vi "Calculator.vi"() -> ()   [LabVIEW 2014]
doc: "This VI is a fully-functional calculator built in LabVIEW. It demonstrates the following concepts taught in the LabVIEW Basics class.\n\n- Dataflow Programming\n- Modular Programming\n- While Loops\n- Shift Registers\n- Case Structures\n- Functional Global Variables\n- Event-Driven Programming\n- VI Documentation\n- Control/Indicator Documentation\n- Custom Controls/Type Definitions\n- LabVIEW Project and Application Builder\n\nAuthor: Erik Johnson, National Instruments"
uses:
  Custom Controls/Operation Buttons.ctl
  Custom Controls/Memory Options.ctl
panel:
  in  "Memory Add":bool
  in  "Memory Store":bool
  in  "Memory Recall":bool
  in  "Memory Clear":bool
  in  "Decimal":bool
  in  "Inverse":bool
  in  "Squared":bool
  in  "Square Root":bool
  in  "Negate":bool
  in  "error in (no error)":errorcluster
  in  "Backspace":bool
  in  "Clear All":bool
  in  "Clear Entry":bool
  in  "Display":ext format="%#_15f"
  in  "Equals":bool
  in  "Divide":bool
  in  "Multiply":bool
  in  "Subtract":bool
  in  "Add":bool
  in  "Zero":bool
  in  "Nine":bool
  in  "Eight":bool
  in  "Seven":bool
  in  "Six":bool
  in  "Five":bool
  in  "Four":bool
  in  "Three":bool
  in  "Two":bool
  in  "One":bool
  # "M"
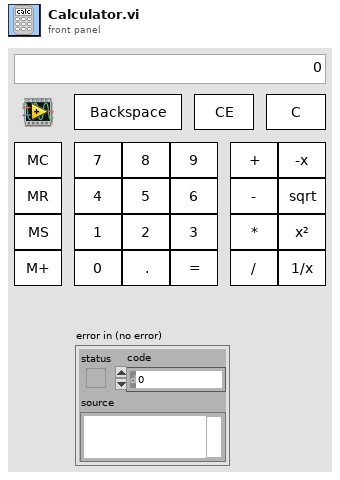
[diagram p1: front panel]
types:
  T1 = typedef "Operation Buttons.ctl" = enum16{"Add", "Subtract", "Multiply", "Divide", "Equals"}
  T2 = typedef "Memory Options.ctl" = enum16{"Memory Clear", "Memory Recall", "Memory Store", "Memory Add"}
  T3 = enum32{"invalid app kind", "Development System", "Run Time System", "Student Edition", "Embedded LabVIEW", "Evaluation", "Custom"}
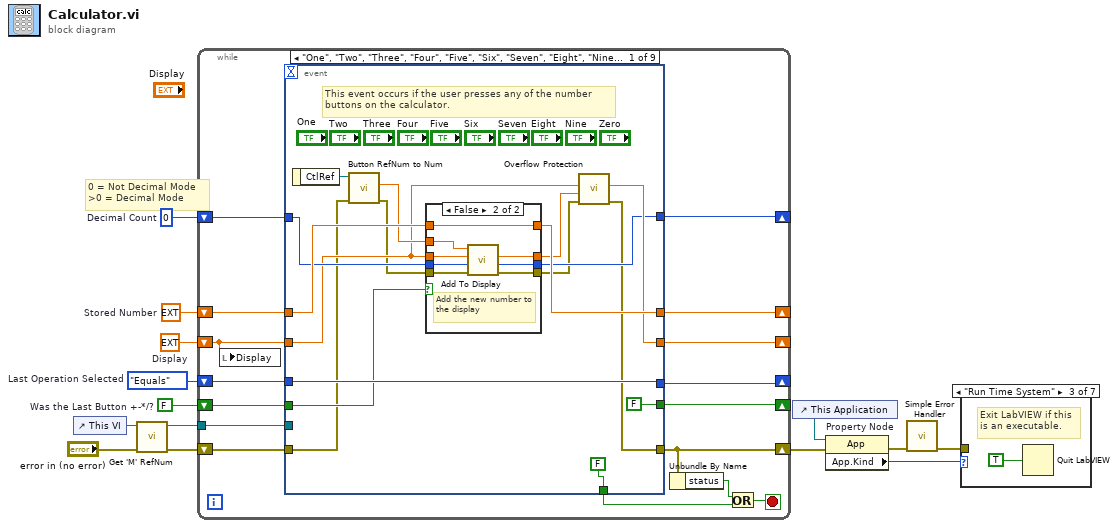
[diagram p0: block diagram]
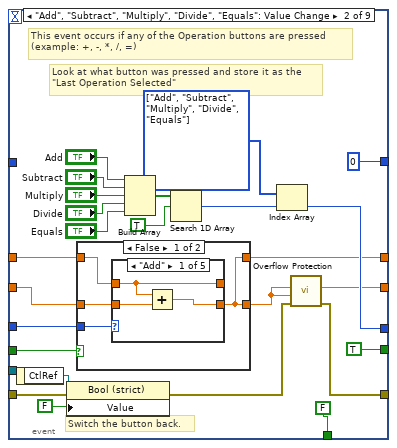
[diagram p9: hidden frame]
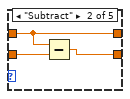
[diagram p10: hidden frame]
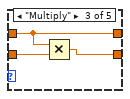
[diagram p11: hidden frame]
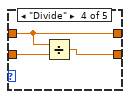
[diagram p12: hidden frame]
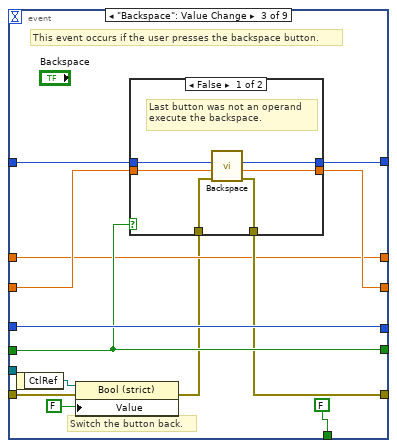
[diagram p15: hidden frame]
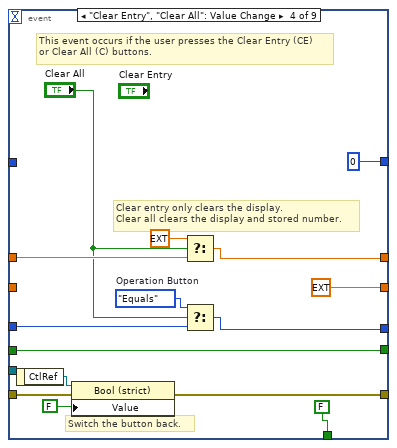
[diagram p17: hidden frame]
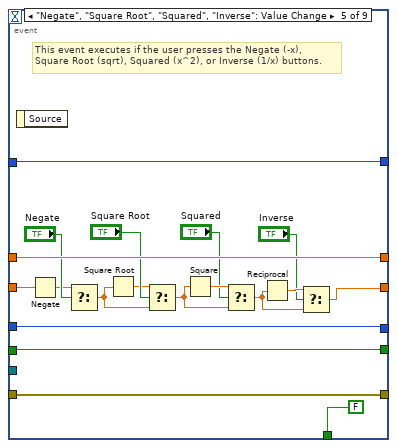
[diagram p18: hidden frame]
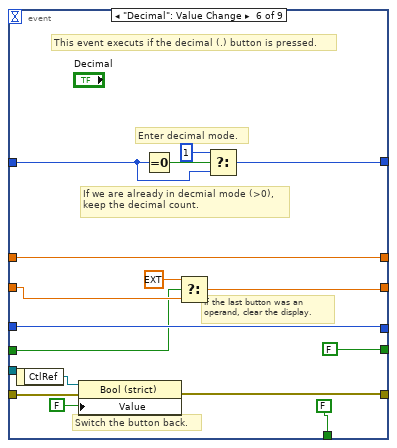
[diagram p19: hidden frame]
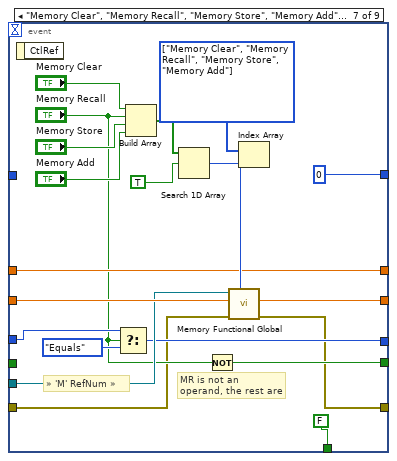
[diagram p20: hidden frame]
diagram:
  w8 = u8 0  # Decimal Count
  w9 = Operation_Buttons."Equals"  # Last Operation Selected
  w12 = FALSE  # Was the Last Button +-*/?
  w13 = ext 0.0  # Stored Number
  w14 = ext 0.0  # Display
  # "0 = Not Decimal Mode\n>0 = Decimal Mode"
  n1 = control-ref of="This VI"() -> (w7:refnum<vi>)
  n2 = call "Get 'M' RefNum.vi"("error in (no error)"="error in (no error)", "This VI"=w7) -> ("error out"=w5:errorcluster, "'M' Refnum"=w6:refnum<vi>)  [unwired: 8 in]
  n3 = while {
    shift-right: [w29] -> _
    shift-left: w14 -> [w30]
    shift-right: [w20] -> _
    shift-left: w13 -> [w28]
    shift-right: [w26] -> _
    shift-left: w9 -> [w27]
    shift-right: [w24] -> _
    shift-left: w12 -> [w25]
    shift-right: [w22] -> _
    shift-left: w8 -> [w23]
    tunnel: w6 -> [w21]
    shift-right: [w17] -> w2
    shift-left: w5 -> [w19]
    stop <- w18 stop-if-true
    n4 = local write "Display"(w30) -> ()
    n5 = event shown="[0] \"One\", \"Two\", \"Three\", \"Four\", \"Five\", \"Six\", \"Seven\", \"Eight\", \"Nine\", \"Zero\": Value Change" {
      selector: _ -> [_ _ _ _ _ _ _ _ _]
      dyn-events: _ -> [_ _ _ _ _ _ _ _ _]
      timeout: _ -> [_ _ _ _ _ _ _ _ _]
      tunnel: [w44 w63 w115 ext 0.0 ("Display") w148 w163 w189 w201 0.0 ("Display")] -> w29
      tunnel: w30 -> [w38 w83 w116 _ w156 w164 w190 w201 _]
      tunnel: [FALSE ("Discard?") FALSE ("Discard?") FALSE ("Discard?") FALSE ("Discard?") FALSE ("Discard?") FALSE ("Discard?") FALSE ("Discard?") FALSE ("Discard?") TRUE ("Discard?")] -> w15
      tunnel: w28 -> [w43 w84 w109 w138 w160 w175 w188 w202 _]
      tunnel: [w45 w62 w109 w137 w160 w175 w188 w202 ext 0.0 ("Stored Number")] -> w20
      tunnel: w27 -> [w37 w74 w117 w132 w159 w176 w185 w205 _]
      tunnel: [w37 w66 w117 w131 w159 w176 w182 w205 w268] -> w26
      tunnel: w25 -> [w36 w72 w114 w141 w144 w161 _ w206 _]
      tunnel: [FALSE ("Discard?") TRUE ("Discard?") w114 w141 w144 FALSE ("Discard?") w180 w206 FALSE ("Discard?")] -> w24
      tunnel: w23 -> [w42 _ w113 _ w143 w173 _ w203 _]
      tunnel: [w41 u8 0 ("Decimal Count") w112 u8 0 ("Decimal Count") w143 w171 u8 0 ("Decimal Count") w203 u8 0 ("Decimal Count")] -> w22
      tunnel: w21 -> [_ _ _ _ _ _ w186 _ _]
      tunnel: w19 -> [w35 w67 w108 w129 w142 w168 w178 w199 w266]
      tunnel: [w32 w60 w110 w128 w142 w167 w177 w198 w266] -> w17
      event "One", "Two", "Three", "Four", "Five", "Six", "Seven", "Eight", "Nine", "Zero": Value Change {
        # "This event occurs if the user presses any of the number\nbuttons on the calculator."
        n6 = event-data() -> ("CtlRef"=w31:refnum<vi>)  [unwired: 1 in]
        n7 = call "Button RefNum to Num.vi"("error in (no error)"=w35, "Button Reference"=w31) -> ("error out"=w34:errorcluster, "Number on Button"=w40:dbl)  [unwired: 8 in]
        n8 = case shown="False" w36 {
          tunnel: w38 -> [w51 w55]
          tunnel: [w49 w54] -> w39
          tunnel: w43 -> [_ w59]
          tunnel: [w51 w59] -> w45
          tunnel: w42 -> [w50 w57]
          tunnel: [w50 w58] -> w41
          tunnel: w40 -> [w49 w56]
          tunnel: w34 -> [w48 w53]
          tunnel: [w48 w52] -> w33
          frame True {
            # "Last button was an operand, refresh the display."
          }
          frame False {
            # "Add the new number to the display"
            n9 = call "Add To Display.vi"("error in (no error)"=w53, "Decimal Count In"=w57, "Display In"=w55, "Number In"=w56) -> ("error out"=w52:errorcluster, "Decimal Count Out"=w58:u8, "Display Out"=w54:ext)  [unwired: 5 in]
          }
        }
        n10 = call "Overflow Protection.vi"("error in (no error)"=w33, "Display After"=w39, "Display Before"=w38) -> ("error out"=w32:errorcluster, "Display Output"=w44:ext)  [unwired: 7 in]
      }
      event "Add", "Subtract", "Multiply", "Divide", "Equals": Value Change {
        w71 = T1[] [enum."Add", enum."Subtract", enum."Multiply", enum."Divide", enum."Equals"] items=["Add", "Subtract", "Multiply", "Divide", "Equals"]
        # "Switch the button back."
        # "Look at what button was pressed and store it as the\n\"Last Operation Selected\""
        # "This event occurs if any of the Operation buttons are pressed\n(example: +, -, *, /, =)"
        n11 = event-data() -> ("CtlRef"=w69:refnum<vi>)  [unwired: 1 in]
        n12 = property class="Bool (strict)"(reference=w69, error in=w67, "Value"=FALSE) -> (error out=w61:errorcluster)  [unwired: 1 out]
        n13 = case shown="False" w72 {
          tunnel: w84 -> [w88 w103]
          tunnel: w83 -> [w87 w104]
          tunnel: w74 -> [w85 _]
          tunnel: [w86 w104] -> w64
          tunnel: [w86 w103] -> w62
          frame False {
            n14 = case shown="\"Add\"" w85 {
              tunnel: w88 -> [w89 w92 w95 w98 w101]
              tunnel: w87 -> [w91 w94 w97 w100 w102]
              tunnel: [w90 w93 w96 w99 w102] -> w86
              tunnel: [w89 w92 w95 w98 w101] -> _
              frame "Add" {
                n15 = Add(x=w89, y=w91) -> (x+y=w90:ext)
              }
              frame "Subtract" {
                n16 = Subtract(x=w92, y=w94) -> (x-y=w93:ext)
              }
              frame "Multiply" {
                n17 = Multiply(x=w95, y=w97) -> (x*y=w96:ext)
              }
              frame "Divide" {
                n18 = Divide(x=w98, y=w100) -> (x/y=w99:ext)
              }
              frame "Equals", Default {
              }
            }
          }
          frame True {
            # "If the last button was an operation, overwrite it and throw out the previous operation."
          }
        }
        n19 = Build Array "Build Array"("Add", "Subtract", "Multiply", "Divide", "Equals") -> (w77:bool[])
        n20 = Search 1D Array(1D array=w77, element=TRUE) -> (index of element=w75:i32)  [unwired: 1 in]
        n21 = Index Array "Index Array"(array=w71, index=w75) -> (element=w66:T1)
        n22 = call "Overflow Protection.vi"("error in (no error)"=w61, "Display After"=w64, "Display Before"=w64) -> ("error out"=w60:errorcluster, "Display Output"=w63:ext)  [unwired: 7 in]
      }
      event "Backspace": Value Change {
        # "Switch the button back."
        # "This event occurs if the user presses the backspace button."
        n23 = event-data() -> ("CtlRef"=w106:refnum<vi>)  [unwired: 1 in]
        n24 = property class="Bool (strict)"(reference=w106, error in=w108, "Value"=FALSE) -> (error out=w107:errorcluster)  [unwired: 1 out]
        n25 = case shown="False" w114 {
          tunnel: w116 -> [w122 w126]
          tunnel: [w120 w126] -> w115
          tunnel: w113 -> [w123 w125]
          tunnel: [w121 w125] -> w112
          tunnel: w107 -> [w119 w124]
          tunnel: [w118 w124] -> w110
          frame False {
            # "Last button was not an operand\nexecute the backspace."
            n26 = call "Backspace.vi"("error in (no error)"=w119, "Display In"=w122, "Decimal Count In"=w123) -> ("error out"=w118:errorcluster, "Display Out"=w120:ext, "Decimal Count Out"=w121:u8)  [unwired: 6 in]
          }
          frame True {
            # "Last button was an operand,\nno need to delete anything."
          }
        }
      }
      event "Clear Entry", "Clear All": Value Change {
        w134 = Operation_Buttons."Equals"  # Operation Button
        # "Switch the button back."
        # "Clear entry only clears the display.\nClear all clears the display and stored number."
        # "This event occurs if the user presses the Clear Entry (CE)\nor Clear All (C) buttons."
        n27 = event-data() -> ("CtlRef"=w130:refnum<vi>)  [unwired: 1 in]
        n28 = property class="Bool (strict)"(reference=w130, error in=w129, "Value"=FALSE) -> (error out=w128:errorcluster)  [unwired: 1 out]
        n29 = Select(t=ext 0.0, s="Clear All", f=w138) -> (s? t:f=w137:ext)
        n30 = Select(t=w134, s="Clear All", f=w132) -> (s? t:f=w131:T1)
      }
      event "Negate", "Square Root", "Squared", "Inverse": Value Change {
        # "This event executes if the user presses the Negate (-x),\nSquare Root (sqrt), Squared (x^2), or Inverse (1/x) buttons."
        n31 = event-data() -> ()  [unwired: 1 in, 1 out]
        n32 = Negate(x=w156) -> (-x=w157:ext)
        n33 = Select(t=w157, s="Negate", f=w156) -> (s? t:f=w154:ext)
        n34 = Square Root(x=w154) -> (sqrt(x)=w153:ext)
        n35 = Select(t=w153, s="Square Root", f=w154) -> (s? t:f=w151:ext)
        n36 = Square(x=w151) -> (x^2=w152:ext)
        n37 = Select(t=w152, s="Squared", f=w151) -> (s? t:f=w147:ext)
        n38 = Reciprocal(x=w147) -> (1/x=w149:ext)
        n39 = Select(t=w149, s="Inverse", f=w147) -> (s? t:f=w148:ext)
      }
      event "Decimal": Value Change {
        # "If the last button was an operand, clear the display."
        # "Switch the button back."
        # "Enter decimal mode."
        # "If we are already in decmial mode (>0),\nkeep the decimal count."
        # "This event executs if the decimal (.) button is pressed."
        n40 = event-data() -> ("CtlRef"=w166:refnum<vi>)  [unwired: 1 in]
        n41 = property class="Bool (strict)"(reference=w166, error in=w168, "Value"=FALSE) -> (error out=w167:errorcluster)  [unwired: 1 out]
        n42 = Equal To 0?(x=w173) -> (x = 0?=w174:bool)
        n43 = Select(t=ext 0.0, s=w161, f=w164) -> (s? t:f=w163:ext)
        n44 = Select(t=u8 1, s=w174, f=w173) -> (s? t:f=w171:u8)
      }
      event "Memory Clear", "Memory Recall", "Memory Store", "Memory Add": Value Change {
        w192 = T2[] [enum."Memory Clear", enum."Memory Recall", enum."Memory Store", enum."Memory Add"] items=["Memory Clear", "Memory Recall", "Memory Store", "Memory Add"]
        # "MR is not an operand, the rest are"
        # "» 'M' RefNum »"
        n45 = event-data() -> ()  [unwired: 1 in, 1 out]
        n46 = Select(t=w185, s="Memory Recall", f=Operation_Buttons."Equals" ("Operation Button")) -> (s? t:f=w182:T1)
        n47 = Build Array "Build Array"("Memory Clear", "Memory Recall", "Memory Store", "Memory Add") -> (w193:bool[])
        n48 = Search 1D Array(1D array=w193, element=TRUE) -> (index of element=w194:i32)  [unwired: 1 in]
        n49 = Not(x="Memory Recall") -> (.not. x?=w180:bool)
        n50 = Index Array "Index Array"(array=w192, index=w194) -> (element=w191:T2)
        n51 = call "Memory Functional Global.vi"("Memory Option"=w191, "error in (no error)"=w178, "Number In"=w190, "'M' Refnum"=w186) -> ("error out"=w177:errorcluster, "Number Out"=w189:ext)  [unwired: 6 in]
      }
      event Key Down? {
        # "This event occurs when a key is pressed.  It then generates a programmatic event using the Value (Signaling) Property Node to trigger the correct event within the program."
        n52 = event-data() -> ("Char"=w200:i16)  [unwired: 1 in]
        n53 = case shown="-1, Default" w200 {
          tunnel: w199 -> [w208 w210 w213 w217 w220 w223 w226 w229 w232 w235 w238 w241 w244 w247 w250 w253 w256 w259 w262 w265]
          tunnel: [w208 w209 w212 w215 w218 w222 w225 w228 w231 w234 w237 w240 w243 w246 w249 w252 w255 w257 w261 w264] -> w198
          frame -1, Default {
          }
          frame 48 {
            n54 = property on="Zero" class="Bool (strict)"(error in=w210, "Val(Sgnl)"=TRUE ("Discard?")) -> (error out=w209:errorcluster)  [unwired: 1 in, 1 out]
          }
          frame 49 {
            n55 = property on="One" class="Bool (strict)"(error in=w213, "Val(Sgnl)"=TRUE ("Discard?")) -> (error out=w212:errorcluster)  [unwired: 1 in, 1 out]
          }
          frame 50 {
            n56 = property on="Two" class="Bool (strict)"(error in=w217, "Val(Sgnl)"=TRUE ("Discard?")) -> (error out=w215:errorcluster)  [unwired: 1 in, 1 out]
          }
          frame 51 {
            n57 = property on="Three" class="Bool (strict)"(error in=w220, "Val(Sgnl)"=TRUE ("Discard?")) -> (error out=w218:errorcluster)  [unwired: 1 in, 1 out]
          }
          frame 52 {
            n58 = property on="Four" class="Bool (strict)"(error in=w223, "Val(Sgnl)"=TRUE ("Discard?")) -> (error out=w222:errorcluster)  [unwired: 1 in, 1 out]
          }
          frame 53 {
            n59 = property on="Five" class="Bool (strict)"(error in=w226, "Val(Sgnl)"=TRUE ("Discard?")) -> (error out=w225:errorcluster)  [unwired: 1 in, 1 out]
          }
          frame 54 {
            n60 = property on="Six" class="Bool (strict)"(error in=w229, "Val(Sgnl)"=TRUE ("Discard?")) -> (error out=w228:errorcluster)  [unwired: 1 in, 1 out]
          }
          frame 55 {
            n61 = property on="Seven" class="Bool (strict)"(error in=w232, "Val(Sgnl)"=TRUE ("Discard?")) -> (error out=w231:errorcluster)  [unwired: 1 in, 1 out]
          }
          frame 56 {
            n62 = property on="Eight" class="Bool (strict)"(error in=w235, "Val(Sgnl)"=TRUE ("Discard?")) -> (error out=w234:errorcluster)  [unwired: 1 in, 1 out]
          }
          frame 57 {
            n63 = property on="Nine" class="Bool (strict)"(error in=w238, "Val(Sgnl)"=TRUE ("Discard?")) -> (error out=w237:errorcluster)  [unwired: 1 in, 1 out]
          }
          frame 43 {
            n64 = property on="Add" class="Bool (strict)"(error in=w241, "Val(Sgnl)"=TRUE ("Discard?")) -> (error out=w240:errorcluster)  [unwired: 1 in, 1 out]
          }
          frame 45 {
            n65 = property on="Subtract" class="Bool (strict)"(error in=w244, "Val(Sgnl)"=TRUE ("Discard?")) -> (error out=w243:errorcluster)  [unwired: 1 in, 1 out]
          }
          frame 42 {
            n66 = property on="Multiply" class="Bool (strict)"(error in=w247, "Val(Sgnl)"=TRUE ("Discard?")) -> (error out=w246:errorcluster)  [unwired: 1 in, 1 out]
          }
          frame 47 {
            n67 = property on="Divide" class="Bool (strict)"(error in=w250, "Val(Sgnl)"=TRUE ("Discard?")) -> (error out=w249:errorcluster)  [unwired: 1 in, 1 out]
          }
          frame 0 {
            # "Press 'Enter'"
            n68 = property on="Equals" class="Bool (strict)"(error in=w253, "Val(Sgnl)"=TRUE ("Discard?")) -> (error out=w252:errorcluster)  [unwired: 1 in, 1 out]
          }
          frame 46 {
            n69 = property on="Decimal" class="Bool (strict)"(error in=w256, "Val(Sgnl)"=TRUE ("Discard?")) -> (error out=w255:errorcluster)  [unwired: 1 in, 1 out]
          }
          frame 8 {
            n70 = property on="Backspace" class="Bool (strict)"(error in=w259, "Val(Sgnl)"=TRUE ("Discard?")) -> (error out=w257:errorcluster)  [unwired: 1 in, 1 out]
          }
          frame 101 {
            # "Press 'E'"
            n71 = property on="Clear Entry" class="Bool (strict)"(error in=w262, "Val(Sgnl)"=TRUE ("Discard?")) -> (error out=w261:errorcluster)  [unwired: 1 in, 1 out]
          }
          frame 99 {
            # "Press 'C'"
            n72 = property on="Clear All" class="Bool (strict)"(error in=w265, "Val(Sgnl)"=TRUE ("Value (Signaling)")) -> (error out=w264:errorcluster)  [unwired: 1 in, 1 out]
          }
        }
        n73 = event-data("Discard?"=TRUE) -> ()  [unwired: 1 in, 1 out]
      }
      event Panel Close? {
        w268 = Operation_Buttons."Equals"  # Operation Button
        # "This event occurs if the user closes the panel."
        n74 = event-data() -> ()  [unwired: 1 in, 1 out]
        n75 = event-data("Discard?"=TRUE) -> ()  [unwired: 1 in, 1 out]
      }
    }
    n76 = Unbundle By Name(w17) -> ("status"=w16:bool)
    n77 = Or(x=w16, y=w15) -> (x .or. y?=w18:bool)
  }
  n78 = control-ref of="This Application"() -> (w11:refnum<vi>)
  n79 = property on="Property Node" class="App"(reference=w11, error in=w2) -> (error out=w4:errorcluster, "App.Kind"=w10:T3)  [unwired: 1 out]
  n80 = call <vilib>:"Simple Error Handler.vi"("error in (no error)"=w4) -> ("error out"=w3:errorcluster)  [unwired: 4 in, 4 out]
  n81 = case shown="\"Run Time System\"" w10 {
    tunnel: w3 -> [_ _ _ _ _ _ _]
    frame "invalid app kind", Default {
    }
    frame "Development System" {
    }
    frame "Run Time System" {
      # "Exit LabVIEW if this\nis an executable."
      n82 = Quit LabVIEW(quit? (T)=TRUE) -> ()
    }
    frame "Student Edition" {
    }
    frame "Embedded LabVIEW" {
    }
    frame "Evaluation" {
    }
    frame "Custom" {
    }
  }
